vi "Test Read.vi"() -> ()   [LabVIEW 2022 SP3, in "Test.lvlib"]
uses:
  Test.lvlib
  <vilib>/IlluminatedG/IG Conditum/Conditum/Entity ID.ctl
  User/Values.ctl
  Conditum SQLite/SQLite/SQLite.lvclass
  C:/Program Files (x86)/National Instruments/LabVIEW 2022/vi.lib/IlluminatedG/IG Conditum/Conditum/Database Platform/Database Platform.lvclass
  User/User.lvclass
  C:/Program Files (x86)/National Instruments/LabVIEW 2022/vi.lib/IlluminatedG/IG Conditum/Conditum/Entity/Entity.lvclass
  <vilib>/IlluminatedG/IG Conditum/Conditum/Entity Manager/Entity Manager.lvclass/Entity Manager.ctl
  User/User.lvclass/User.ctl
  <vilib>/IlluminatedG/IG Conditum/Conditum/Columns/String/String.lvclass/String.ctl
  <vilib>/IlluminatedG/IG Conditum/Conditum/Columns/Timestamp/Timestamp.lvclass/Timestamp.ctl
  <vilib>/IlluminatedG/IG Conditum/Conditum/Columns/Boolean/Boolean.lvclass/Boolean.ctl
  <vilib>/IlluminatedG/IG Conditum/Conditum/Columns/Integer/Integer.lvclass/Integer.ctl
  <vilib>/IlluminatedG/IG Conditum/Conditum/Columns/String/Get.vi
  <vilib>/IlluminatedG/IG Conditum/Conditum/Columns/Timestamp/Get.vi
  <vilib>/IlluminatedG/IG Conditum/Conditum/Columns/Boolean/Get.vi
  <vilib>/IlluminatedG/IG Conditum/Conditum/Columns/Integer/Get.vi
  <vilib>/IlluminatedG/IG Conditum/Conditum/Entity Manager/Entity Manager.lvclass
  C:/dev/lv/illuminated-g/lv-conditum-sqlite/Conditum SQLite/SQLite/SQLite.lvclass
  C:/dev/lv/illuminated-g/lv-conditum-sqlite/Test/User/User.lvclass
  <vilib>/IlluminatedG/IG Conditum/Conditum/Conditum.lvlib
panel:
  out "Values":T1
  in  "Entity ID":T2
  out "error out":errorcluster
  in  "DB Path":path=path "C:/dev/lv/illuminated-g/lv-conditum-sqlite/Test/test.db"
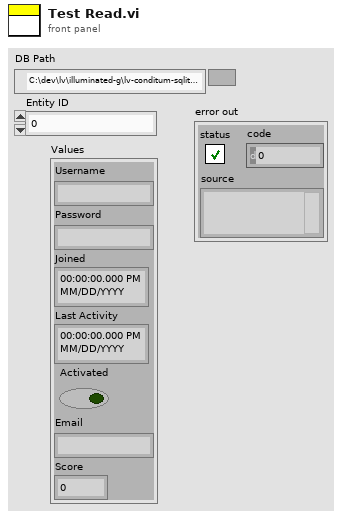
[diagram p1: front panel]
types:
  T1 = typedef "Test.lvlib/User.lvclass/Values.ctl" = cluster{"Username":string, "Password":string, "Joined":timestamp, "Last Activity":timestamp, "Activated":bool, "Email":string, "Score":i64}
  T2 = typedef "Conditum.lvlib/Entity ID.ctl" = i64
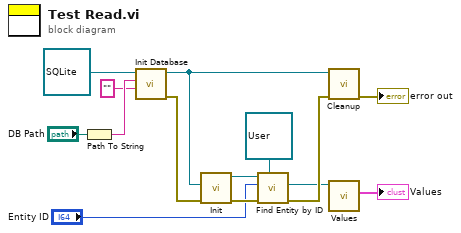
[diagram p0: block diagram]
diagram:
  n1 = Path To String(path="DB Path") -> (string=w12:string)
  n2 = call-dynamic "Init Database.vi"("Database"="", "Resource"=w12, "Database in"=refnum<class "SQLite.lvclass"> refnum) -> ("error out"=w4:errorcluster, "Database out"=w5:refnum<class "SQLite.lvclass">)  [unwired: 7 in]
  n3 = call <vilib>:"Init.vi"("error in (no error)"=w4, "Database"=w5) -> ("error out"=w6:errorcluster, "Entity Manager out"=w7:refnum<class "Entity Manager.lvclass">)  [unwired: 8 in]
  n4 = call <vilib>:"Find Entity by ID.vi"("Entity Type"=refnum<class "User.lvclass"> refnum ("Test.lvlib:User.lvclass"), "error in (no error)"=w6, "Entity ID"="Entity ID", "Entity Manager in"=w7) -> ("error out"=w14:errorcluster, "Entity"=w2:refnum<class "User.lvclass">)  [unwired: 5 in, 1 out]
  n5 = call-dynamic "Cleanup.vi"("error in (no error)"=w14, "SQLite in"=w5) -> ("error out"=→"error out":errorcluster)  [unwired: 9 in]
  n6 = call "Values.vi"("User in"=w2) -> ("Values"=→"Values":T1)  [unwired: 10 in]
